vi "CD Read Engine_Parse Message_Update Channels.vi"(6 "Broadcast?":bool, 8 "error in (no error)":errorcluster, 9 "NORESP?":bool, 10 "Frame Descriptor":T2 {"RT"."Status Channel Ref" format="%.0x"; "RT"."Words Block Data Refs"."Data Reference" format="%.0x"; "RT"."Timestamp Channel Data Reference" format="%.0x"; "BC"."Status Channel Refs" format="%.0x"; "BC"."Words Block Data Refs"."Data Reference" format="%.0x"; "BC"."Timestamp Channel Data Reference" format="%.0x"}, 11 "record in":T1 {"type" format="%04x"; "activity" format="%04x"; "error" format="%04x"; "cwd1" format="%04x"; "cwd2" format="%04x"; "swd1" format="%04x"; "swd2" format="%04x"; "data" format="%04x"}) -> (0 "error out":errorcluster, 1 "Valid Frame?":bool, 3 "Timestamp (s)":dbl)   [LabVIEW 2020, in "Ballard MIL-1553 Engine.lvlib"]
uses:
  Ballard MIL-1553 Engine.lvlib
  Controls/RT Inline Frame Descriptor.ctl
  Controls/RT Inline Frame Descriptor_BC.ctl
  <vilib>/NI VeriStand/Custom Device API/Data Reference.ctl
  <vilib>/NI VeriStand/Custom Device API/Block Data Reference.ctl
  <vilib>/NI VeriStand/Custom Device API/Custom Device Item Ref.ctl
  Controls/RT Inline Frame Descriptor_RT.ctl
  Shared/Controls and Global/RT CWD2.ctl
  Shared/Controls and Global/RT CWD1.ctl
  Shared/Controls and Global/RT messageType.ctl
  <instrlib>/BTICardLib/Public/Controls/1553 Record.ctl
  <vilib>/NI VeriStand/Custom Device API/Global Data Refs.vi
  <vilib>/NI VeriStand/Custom Device API/Custom Device API.lvlib
  Shared/Ballard 1553 Shared.lvlib
  <vilib>/NI VeriStand/Custom Device Tools/Custom Device Utility Library/Custom Device Utility Library.lvlib
  <instrlib>/BTICardLib/BTICardLV.lvlib
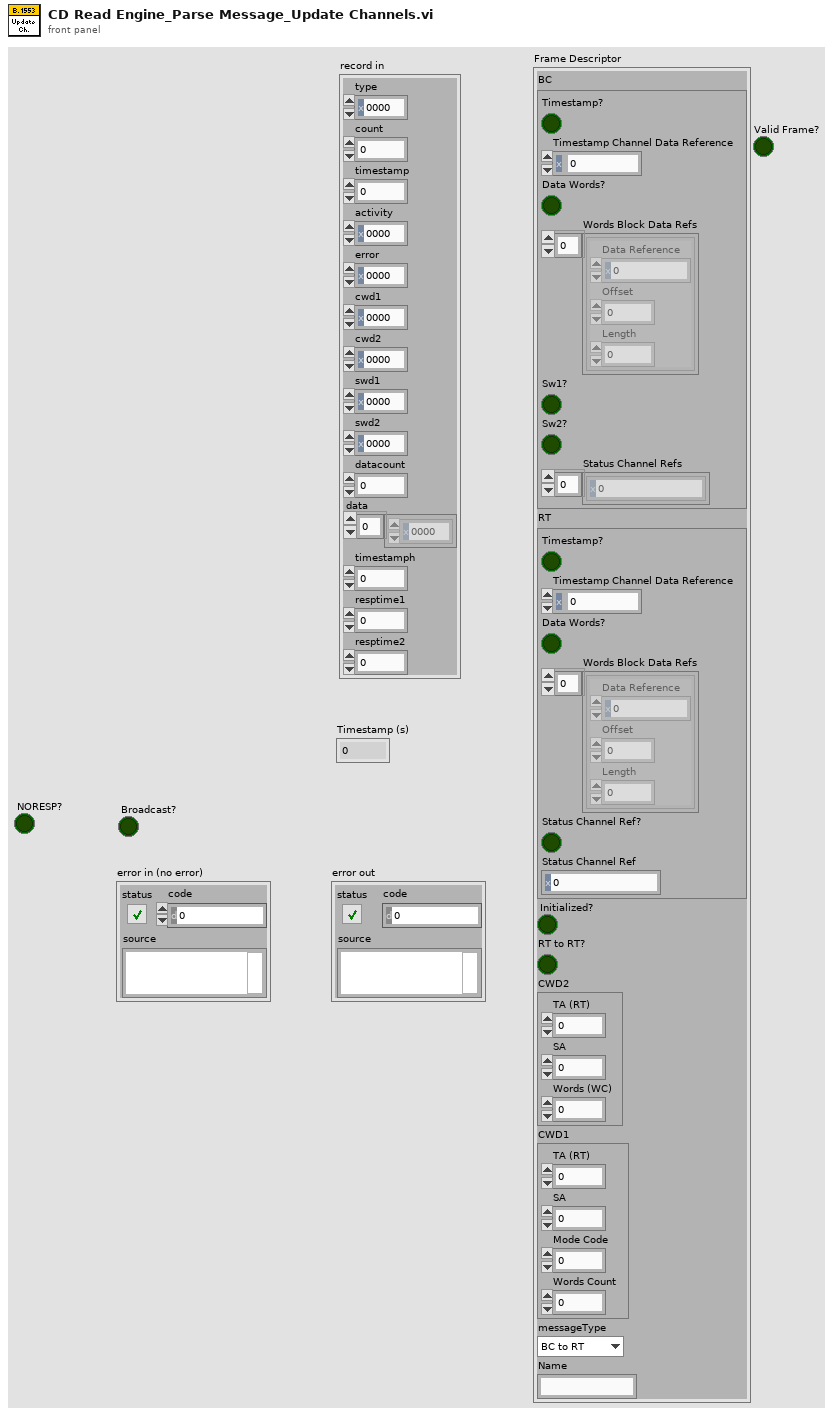
[diagram p1: front panel]
types:
  T1 = typedef "BTICardLV.lvlib/1553 Record.ctl" = cluster{"type":u16, "count":u16, "timestamp":u32, "activity":u16, "error":u16, "cwd1":u16, "cwd2":u16, "swd1":u16, "swd2":u16, "datacount":u16, "data":u16[], "timestamph":u32, "resptime1":u16, "resptime2":u16}
  T2 = typedef "Ballard MIL-1553 Engine.lvlib/RT Inline Frame Descriptor.ctl" = cluster{"BC":T3, "RT":T7, "Initialized?":bool, "RT to RT?":bool, "CWD2":T8, "CWD1":T9, "messageType":T10, "Name":string}
  T3 = typedef "Ballard MIL-1553 Engine.lvlib/RT Inline Frame Descriptor_BC.ctl" = cluster{"Timestamp?":bool, "Timestamp Channel Data Reference":T4, "Data Words?":bool, "Words Block Data Refs":T5[], "Sw1?":bool, "Sw2?":bool, "Status Channel Refs":T6[]}
  T4 = typedef "Custom Device API.lvlib/Data Reference.ctl" = i32
  T5 = typedef "Custom Device API.lvlib/Block Data Reference.ctl" = cluster{"Data Reference":T4, "Offset":u64, "Length":u64}
  T6 = typedef "Custom Device API.lvlib/Custom Device Item Ref.ctl" = u64
  T7 = typedef "Ballard MIL-1553 Engine.lvlib/RT Inline Frame Descriptor_RT.ctl" = cluster{"Timestamp?":bool, "Timestamp Channel Data Reference":T4, "Data Words?":bool, "Words Block Data Refs":T5[], "Status Channel Ref?":bool, "Status Channel Ref":T6}
  T8 = typedef "Ballard 1553 Shared.lvlib/RT CWD2.ctl" = cluster{"TA (RT)":i8, "SA":i8, "Words (WC)":i8}
  T9 = typedef "Ballard 1553 Shared.lvlib/RT CWD1.ctl" = cluster{"TA (RT)":i8, "SA":i8, "Mode Code":i8, "Words Count":i8}
  T10 = typedef "Ballard 1553 Shared.lvlib/RT messageType.ctl" = enum16{"BC to RT", "RT to BC", "RT to RT", "MC (Rx)", "MC (Tx)"}
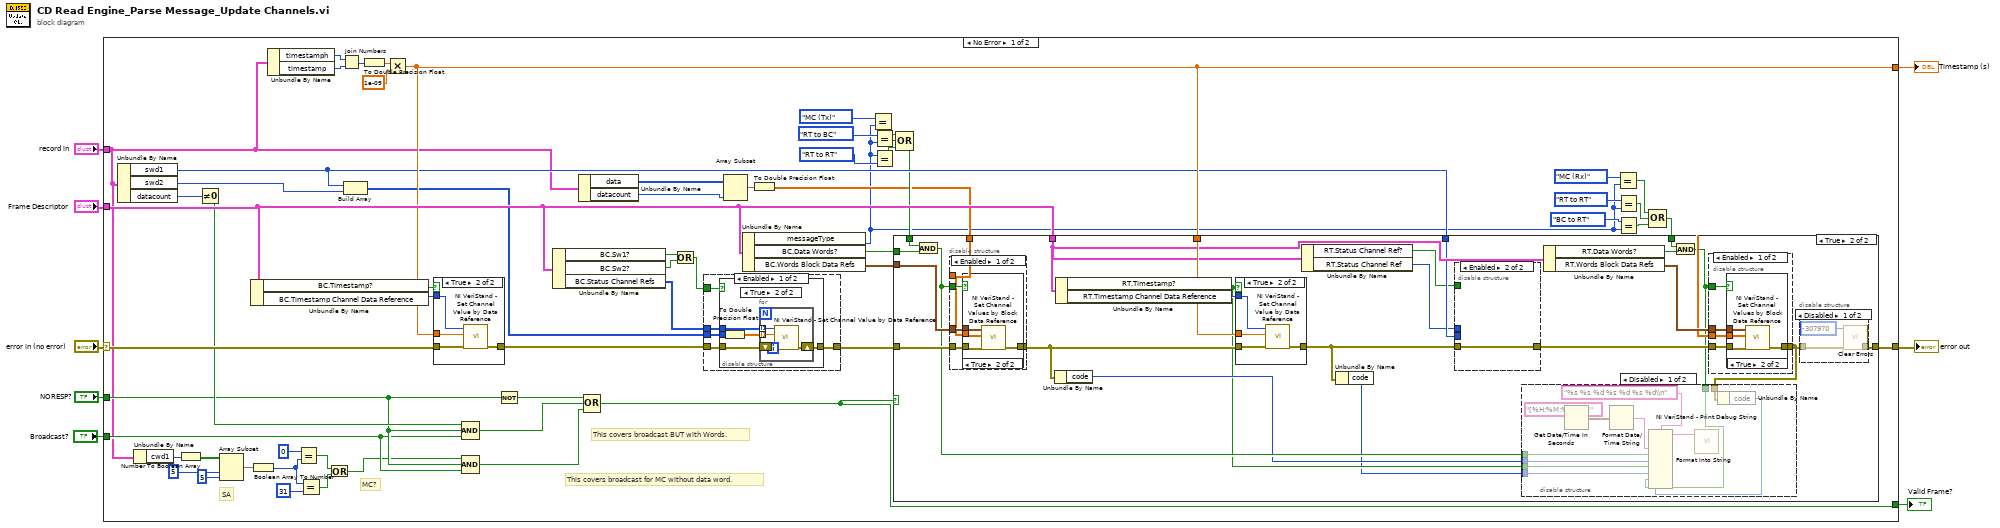
[diagram p0: block diagram]
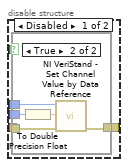
[diagram p9: hidden frame]
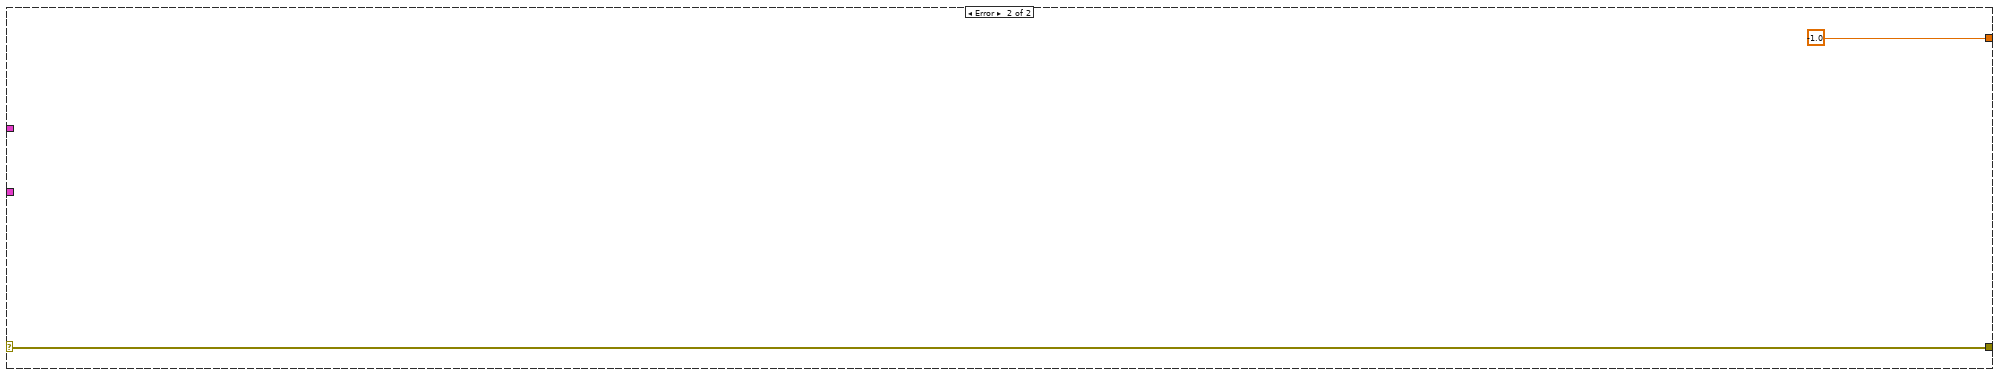
[diagram p15: hidden frame]
diagram:
  n1 = case shown="No Error" "error in (no error)" {
    selector: "error in (no error)" -> [w64 w171]
    tunnel: "Frame Descriptor" -> [w63 _]
    tunnel: [w61 w171] -> w7
    tunnel: "record in" -> [w24 _]
    tunnel: "NORESP?" -> [w26 _]
    tunnel: [w62 -1.0] -> w3
    tunnel: "Broadcast?" -> [w25 _]
    tunnel: [w12 _] -> w1
    frame No Error {
      # "SA"
      # "MC?"
      # "This covers broadcast for MC without data word."
      # "This covers broadcast BUT with Words."
      n2 = Unbundle By Name(w24) -> ("swd1"=w55:u16, "swd2"=w57:u16, "datacount"=w28:u16)
      n3 = Unbundle By Name(w24) -> ("cwd1"=w20:u16)
      n4 = Number To Boolean Array(number=w20) -> (Boolean array=w19:bool[])
      n5 = Not Equal To 0?(x=w28) -> (x != 0?=w27:bool)
      n6 = Array Subset(array=w19, index=5, length=5) -> (w23:bool[])
      n7 = Unbundle By Name(w63) -> ("BC.Timestamp?"=w60:bool, "BC.Timestamp Channel Data Reference"=w59:T4)
      n8 = Boolean Array To Number(Boolean array=w23) -> (number=w18:u32)
      n9 = Unbundle By Name(w24) -> ("timestamph"=w65:u32, "timestamp"=w66:u32)
      n10 = Equal?(x=u32 0, y=w18) -> (x = y?=w17:bool)
      n11 = Equal?(x=w18, y=u32 31) -> (x = y?=w16:bool)
      n12 = Or(x=w17, y=w16) -> (x .or. y?=w13:bool)
      n13 = Join Numbers(hi=w65, lo=w66) -> ((hi.lo)=w67:u64)
      n14 = Build Array(w55, w57) -> (w56:u16[])
      n15 = To Double Precision Float(number=w67) -> (double precision float=w68:dbl)
      n16 = Multiply(x=w68, y=1e-09) -> (x*y=w62:dbl)
      n17 = case shown="True" w60 {
        tunnel: w59 -> [_ w169]
        tunnel: w62 -> [_ w168]
        tunnel: w64 -> [w165 w167]
        tunnel: [w165 w166] -> w58
        frame False {
        }
        frame True {
          n18 = call <vilib>:"NI VeriStand - Set Channel Value by Data Reference.vi"("error in (no error)"=w167, "Value"=w168, "Data Reference in"=w169) -> ("error out"=w166:errorcluster)  [unwired: 8 in]
        }
      }
      n19 = Compound Arithmetic op=AND(w27, w26, w25) -> (w10:bool)
      n20 = Compound Arithmetic op=AND(w13, w26, w25) -> (w9:bool)
      n21 = Not(x=w26) -> (.not. x?=w11:bool)
      n22 = Unbundle By Name(w63) -> ("BC.Sw1?"=w53:bool, "BC.Sw2?"=w54:bool, "BC.Status Channel Refs"=w51:T6[])
      n23 = Unbundle By Name(w24) -> ("data"=w48:u16[], "datacount"=w35:u16)
      n24 = Compound Arithmetic op=OR(w11, w10, w9) -> (w12:bool)
      n25 = Or(x=w53, y=w54) -> (x .or. y?=w52:bool)
      n26 = disable-structure shown="Enabled" {
        disable-tunnel: w58 -> [w74 w85]
        disable-tunnel: w56 -> [w73 _]
        disable-tunnel: w52 -> [w72 _]
        disable-tunnel: w51 -> [w71 _]
        disable-tunnel: [w70 w85] -> w50
        frame Enabled {
          n27 = case shown="True" w72 {
            tunnel: w71 -> [_ w80]
            tunnel: w73 -> [_ w79]
            tunnel: w74 -> [w75 w78]
            tunnel: [w75 w77] -> w70
            frame False {
            }
            frame True {
              n28 = To Double Precision Float(number=w79) -> (double precision float=w76:dbl[])
              n29 = for {
                tunnel: w80 -> [w84] mode=indexing
                tunnel: w76 -> [w83] mode=indexing
                shift-right: [w81] -> w77
                shift-left: w78 -> [w82]
                n30 = call <vilib>:"NI VeriStand - Set Channel Value by Data Reference.vi"("error in (no error)"=w82, "Value"=w83, "Data Reference in"=w84) -> ("error out"=w81:errorcluster)  [unwired: 8 in]
              }
            }
          }
        }
        frame Disabled {
        }
      }
      n31 = Array Subset(array=w48, length=w35) -> (w47:u16[])  [unwired: 1 in]
      n32 = Unbundle By Name(w63) -> ("messageType"=w29:T10, "BC.Data Words?"=w39:bool, "BC.Words Block Data Refs"=w49:T5[])
      n33 = To Double Precision Float(number=w47) -> (double precision float=w36:dbl[])
      n34 = Equal?(x=RT_messageType."MC (Tx)", y=w29) -> (x = y?=w30:bool)
      n35 = Equal?(x=RT_messageType."RT to BC", y=w29) -> (x = y?=w41:bool)
      n36 = Equal?(x=w29, y=RT_messageType."RT to RT") -> (x = y?=w40:bool)
      n37 = Compound Arithmetic op=OR(w30, w41, w40) -> (w45:bool)
      n38 = Equal?(x=RT_messageType."MC (Rx)", y=w29) -> (x = y?=w32:bool)
      n39 = Equal?(x=RT_messageType."RT to RT", y=w29) -> (x = y?=w38:bool)
      n40 = Equal?(x=RT_messageType."BC to RT", y=w29) -> (x = y?=w37:bool)
      n41 = Compound Arithmetic op=OR(w32, w38, w37) -> (w43:bool)
      n42 = case shown="True" w12 {
        tunnel: w62 -> [_ w110]
        tunnel: [w86 w87] -> w61
        tunnel: w63 -> [_ w109]
        tunnel: w55 -> [_ w108]
        tunnel: w50 -> [w86 w107]
        tunnel: w49 -> [_ w106]
        tunnel: w45 -> [_ w100]
        tunnel: w43 -> [_ w99]
        tunnel: w39 -> [_ w98]
        tunnel: w36 -> [_ w96]
        frame False {
          # "NO RESPONSE from RT."
        }
        frame True {
          n43 = And(x=w100, y=w98) -> (x .and. y?=w95:bool)
          n44 = disable-structure shown="Enabled" {
            disable-tunnel: w95 -> [w153 _]
            disable-tunnel: w107 -> [w152 w159]
            disable-tunnel: w106 -> [w151 _]
            disable-tunnel: [w150 w159] -> w94
            disable-tunnel: w96 -> [w149 _]
            frame Enabled {
              n45 = case shown="True" w153 {
                tunnel: w152 -> [w154 w158]
                tunnel: w151 -> [_ w157]
                tunnel: w149 -> [_ w156]
                tunnel: [w154 w155] -> w150
                frame False {
                }
                frame True {
                  n46 = call <vilib>:"NI VeriStand - Set Channel Values by Block Data Reference.vi"("error in (no error)"=w158, "Values Array in"=w156, "Block Data Ref"=w157) -> ("error out"=w155:errorcluster)  [unwired: 6 in, 2 out]
                }
              }
            }
            frame Disabled {
            }
          }
          n47 = Unbundle By Name(w94) -> ("code"=w92:i32)
          n48 = Unbundle By Name(w109) -> ("RT.Timestamp?"=w91:bool, "RT.Timestamp Channel Data Reference"=w104:T4)
          n49 = case shown="True" w91 {
            tunnel: w104 -> [_ w164]
            tunnel: w110 -> [_ w163]
            tunnel: w94 -> [w160 w162]
            tunnel: [w160 w161] -> w93
            frame False {
            }
            frame True {
              n50 = call <vilib>:"NI VeriStand - Set Channel Value by Data Reference.vi"("error in (no error)"=w162, "Value"=w163, "Data Reference in"=w164) -> ("error out"=w161:errorcluster)  [unwired: 8 in]
            }
          }
          n51 = Unbundle By Name(w109) -> ("RT.Status Channel Ref?"=w102:bool, "RT.Status Channel Ref"=w103:T6)
          n52 = Unbundle By Name(w93) -> ("code"=w90:i32)
          n53 = disable-structure shown="Enabled" {
            disable-tunnel: w108 -> [w141 _]
            disable-tunnel: w103 -> [w140 _]
            disable-tunnel: w102 -> [w139 _]
            disable-tunnel: w93 -> [w138 w148]
            disable-tunnel: [w137 w148] -> w101
            frame Disabled {
              n54 = case shown="True" w139 {
                tunnel: w140 -> [_ w145]
                tunnel: [w142 w146] -> w137
                tunnel: w138 -> [w142 w147]
                tunnel: w141 -> [_ w144]
                frame False {
                }
                frame True {
                  n55 = To Double Precision Float(number=w144) -> (double precision float=w143:dbl)
                  n56 = call <vilib>:"NI VeriStand - Set Channel Value by Data Reference.vi"("error in (no error)"=w147, "Value"=w143, "Data Reference in"=w145) -> ("error out"=w146:errorcluster)  [unwired: 8 in]
                }
              }
            }
            frame Enabled {
            }
          }
          n57 = Unbundle By Name(w109) -> ("RT.Data Words?"=w97:bool, "RT.Words Block Data Refs"=w105:T5[])
          n58 = And(x=w99, y=w97) -> (x .and. y?=w89:bool)
          n59 = disable-structure shown="Enabled" {
            disable-tunnel: [w130 w136] -> w88
            disable-tunnel: w105 -> [w129 _]
            disable-tunnel: w89 -> [w128 _]
            disable-tunnel: w96 -> [w127 _]
            disable-tunnel: w101 -> [w126 w136]
            frame Enabled {
              n60 = case shown="True" w128 {
                tunnel: w126 -> [w131 w135]
                tunnel: w129 -> [_ w134]
                tunnel: [w131 w133] -> w130
                tunnel: w127 -> [_ w132]
                frame False {
                }
                frame True {
                  n61 = call <vilib>:"NI VeriStand - Set Channel Values by Block Data Reference.vi"("error in (no error)"=w135, "Values Array in"=w132, "Block Data Ref"=w134) -> ("error out"=w133:errorcluster)  [unwired: 6 in, 2 out]
                }
              }
            }
            frame Disabled {
            }
          }
          n62 = disable-structure shown="Disabled" {
            disable-tunnel: w95 -> [w121 _]
            disable-tunnel: w92 -> [w120 _]
            disable-tunnel: w91 -> [w119 _]
            disable-tunnel: w90 -> [w118 _]
            disable-tunnel: w89 -> [w117 _]
            disable-tunnel: w88 -> [w115 _]
            frame Disabled {
              (unwired) "[%H:%M:%S%3u]" ("time format string (%c)")
              n63 = Get Date/Time In Seconds() -> (seconds since 1Jan1904=w124:timestamp)
              n64 = Format Date/Time String(seconds (now)=w124) -> (date/time string=w123:string)  [unwired: 2 in]
              n65 = Unbundle By Name(w115) -> ("code"=w116:i32)
              n66 = Format Into String(format string="%s %s %d %s %d %s %d\\n", w123, w121, w120, w119, w118, w117, w116) -> (resulting string=w125:string)  [unwired: 2 in, 1 out]
              n67 = call <vilib>:"NI VeriStand - Print Debug String.vi"("Message"=w125) -> ()  [unwired: 10 in, 1 out]
            }
            frame Enabled {
            }
          }
          n68 = disable-structure shown="Disabled" {
            disable-tunnel: w88 -> [w113 w114]
            disable-tunnel: [w111 w114] -> w87
            frame Disabled {
              n69 = call <vilib>:"Clear Errors.vi"("error in (no error)"=w113, "specific error code to clear (0: all)"=-307970) -> ("error out"=w111:errorcluster)  [unwired: 4 in, 1 out]
            }
            frame Enabled {
            }
          }
        }
      }
    }
    frame Error {
    }
  }
  "error out" <- w7
  "Timestamp (s)" <- w3
  "Valid Frame?" <- w1
